vi "Squeeze group (SubVI).vi"(6 "reset":bool, 7 "Step length":dbl, 8 "Inner bound":dbl, 9 "Outer bound":dbl, 10 "Trap cluster in":T1, 11 "ROI in":T2) -> (3 "output cluster":T1)   [LabVIEW 2012]
uses:
  Trap cluster.ctl
panel:
  out "Current relative pos":dbl
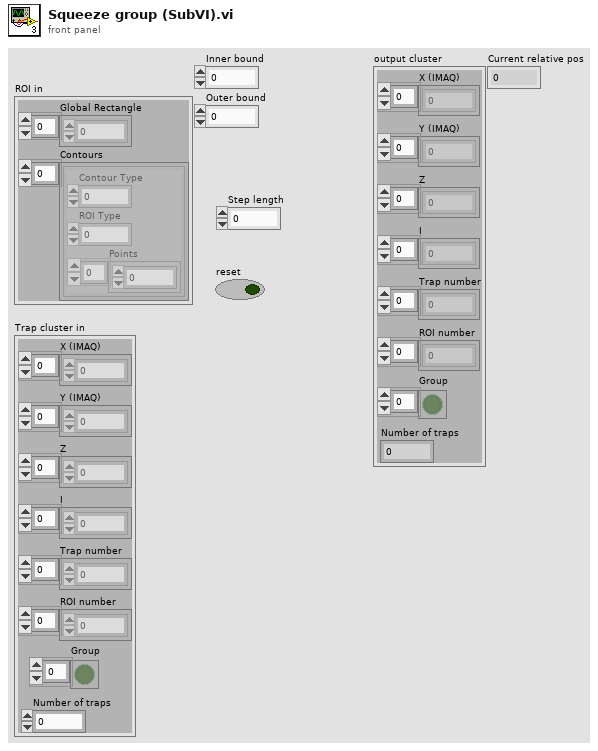
[diagram p1: front panel]
types:
  T1 = typedef "Trap cluster.ctl" = cluster{"X (IMAQ)":sgl[], "Y (IMAQ)":sgl[], "Z":sgl[], "I":sgl[], "Trap number":i32[], "ROI number":i32[], "Number of traps":i32, "Group":bool[]}
  T2 = cluster{"Global Rectangle":i32[], "Contours":cluster{"Contour Type":u32, "ROI Type":u32, "Points":i32[]}[]}
  T3 = cluster{"Contour Type":u32, "ROI Type":u32, "Points":i32[]}[]
  T4 = cluster{"Contour Type":u32, "ROI Type":u32, "Points":i32[]}
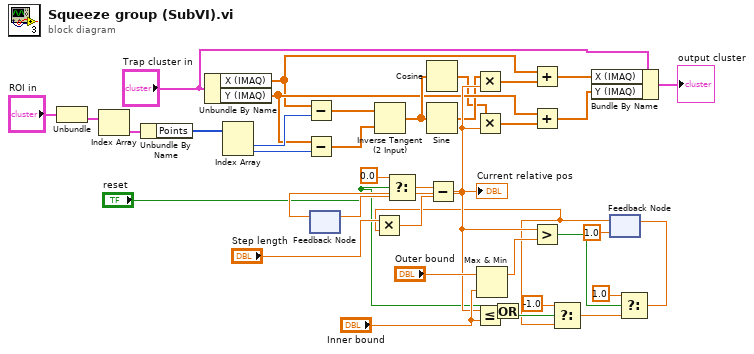
[diagram p0: block diagram]
diagram:
  n1 = Unbundle("ROI in") -> ("Contours"=w35:T3)  [unwired: 1 out]
  n2 = Index Array(array=w35) -> (element=w36:T4)  [unwired: 1 in]
  n3 = Unbundle By Name(w36) -> ("Points"=w37:i32[])
  n4 = Unbundle By Name("Trap cluster in") -> ("X (IMAQ)"=w7:sgl[], "Y (IMAQ)"=w8:sgl[])
  n5 = Index Array(array=w37) -> (element #1=w34:i32, element #2=w33:i32)  [unwired: 2 in]
  n6 = Subtract(x=w7, y=w34) -> (x-y=w32:sgl[])
  n7 = Subtract(x=w8, y=w33) -> (x-y=w31:sgl[])
  n8 = feedback #1() -> (w20:dbl)  [unwired: 1 in]
  n9 = Inverse Tangent (2 Input)(1:w31, 2:w32) -> (0:w30:sgl[])
  n10 = Select(t=0.0, s="reset", f=w20) -> (s? t:f=w21:dbl)
  n11 = Cosine(x=w30) -> (cos(x)=w1:sgl[])
  n12 = Sine(x=w30) -> (sin(x)=w2:sgl[])
  n13 = Max & Min(x="Outer bound", y="Inner bound") -> (max(x,y)=w18:dbl)  [unwired: 1 out]
  n14 = feedback #2(1.0 ("t")) -> (w4:dbl)
  n15 = Multiply(x="Step length", y=w4) -> (x*y=w19:dbl)
  n16 = Subtract(x=w21, y=w19) -> (x-y=w9:dbl)
  "Current relative pos" <- w9
  n17 = feedback-in #1(w9) -> ()
  n18 = Multiply(x=w2, y=w9) -> (x*y=w29:dbl[])
  n19 = Multiply(x=w1, y=w9) -> (x*y=w28:dbl[])
  n20 = Less Or Equal?(x=w9, y="Inner bound") -> (x <= y?=w15:bool)
  n21 = Or(x="reset", y=w15) -> (x .or. y?=w6:bool)
  n22 = Add(x=w7, y=w29) -> (x+y=w26:dbl[])
  n23 = Add(x=w8, y=w28) -> (x+y=w25:dbl[])
  n24 = Greater?(x=w9, y=w18) -> (0:w14:bool)
  n25 = Select(t=-1.0, s=w6, f=w4) -> (s? t:f=w11:dbl)
  n26 = Bundle By Name(cluster="Trap cluster in", "X (IMAQ)"=w26, "Y (IMAQ)"=w25) -> (→"output cluster":T1)
  n27 = Select(t=1.0, s=w14, f=w11) -> (s? t:f=w10:dbl)
  n28 = feedback-in #2(w10) -> ()
